vi "Fmt_PrintLineMsg.vi"(10 "Color":u32(colorbox), 11 "LineToPrint":string) -> (3 "<JSON>":string)   [LabVIEW 2020]
uses:
  td/td_PrintLine.ctl
  dc858e2f-0d51-461b-bc00-a79f37a680c9.vi
  <vilib>/JDP Science/JSONtext/Variant to JSON Text.vi
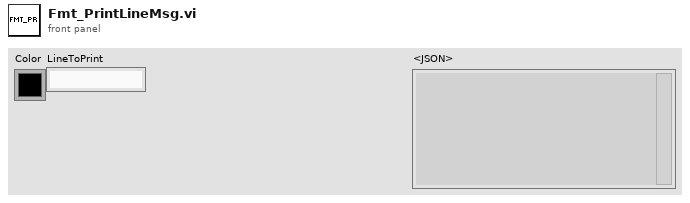
[diagram p1: front panel]
types:
  T1 = typedef "td_PrintLine.ctl" = cluster{"LineToPrint":string, "TxtColor":cluster{"r":u8, "b":u8, "g":u8}}
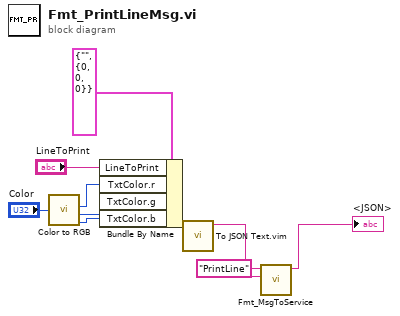
[diagram p0: block diagram]
diagram:
  n1 = call <vilib>:"Color to RGB.vi"("Color"="Color") -> ("R"=w7:u8, "G"=w6:u8, "B"=w5:u8)  [unwired: 1 out]
  n2 = Bundle By Name(cluster=T1 {"LineToPrint"="", "TxtColor"={"r"=0, "b"=0, "g"=0}} ("Cluster"), "LineToPrint"="LineToPrint", "TxtColor.r"=w7, "TxtColor.g"=w6, "TxtColor.b"=w5) -> (w8:T1)
  n3 = call "To JSON Text.vim"("Anything"=w8) -> ("<JSON>"=w2:string)  [unwired: 9 in, 1 out]
  n4 = call "Fmt_MsgToService.vi"("Data"=w2, "state"="PrintLine") -> ("<JSON>"=→"<JSON>":string)  [unwired: 9 in]
